vi "Unicode Tab Page Example.vi"() -> ()   [LabVIEW 2020]
doc: "This example demonstrates how to configure a new tab control to display unicode text."
uses:
  Unicode/Controls/String Encoding.ctl
  Types/UTF-8 String/UTF-8 String.lvclass/UTF-8 String.ctl
  Dialog & User Interface/Polymorphic VIs/Write Control Text/Write Tab Pages (UTF-8 String).vi
  Dialog & User Interface/Polymorphic VIs/Write Control Text/Write String Value (UTF-8 String).vi
  Unicode/Encode String.vi
  Dialog & User Interface/Polymorphic VIs/Write Control Text/Write Tab Pages (UTF-8 String).vi/5206cb6b-04fb-41f5-a37e-29c14f142303.vi
  Dialog & User Interface/Polymorphic VIs/Write Control Text/Write String Value (UTF-8 String).vi/5206cb6b-04fb-41f5-a37e-29c14f142303.vi
  Unicode/Detect String Encoding.vi
  Private/Conversion/Text to UTF-8.vi
  Private/Conversion/Polymorphic VIs/Text to UTF-8 (LabVIEW String).vi
  Private/Conversion/Encoded UTF-8 String to Encoded UTF-16LE String.vi
  Unicode/SubVIs/UTF-16 Byte Swap.vi
  Private/Conversion/UTF-8 to Text.vi
  Private/Conversion/Polymorphic VIs/UTF-8 to Text (LabVIEW String).vi
  Private/Conversion/Encoded UTF-16LE String to Encoded UTF-8 String.vi
  Unicode/Prepend BOM.vi
  Private/Conversion/Text as Encoded String.vi
  Private/Conversion/Polymorphic VIs/Text as Encoded String (UTF-8 String).vi
  Unicode/Strip BOM.vi
  Unicode/Detect String Encoding.vi/f4e2713d-ca87-487a-b901-d606fc3002c3.vi
  Unicode/SubVIs/Byte Order Marks.vi
  Unicode/Detect BOM.vi
  Types/UTF-8 String/Read Encoded UTF-8 String.vi
  Private/Library/gu_is_text_utf16.vi
  Private/Library/gu_is_text_utf8.vi
  Private/User Interface/Write String.vi
  Private/User Interface/Write Tab Control.vi
  Types/UTF-8 String/UTF-8 String.lvclass
  G-Unicode.lvlib
panel:
  in  "Tab Control":enum32{"Page 1", "Page 2", "Page 3", "Page 4"}(tab)
  out "Unicode String":string
  # "This example demonstrates how to configure a new tab control to display unicode text.\n\nWhen a tab control is first created the tab page text is not enabled for unicode display. To enable unicode display each page must first set the Independent Label property to TRUE. Once set, unicode text then needs to be copied over the text of every tab page. Once these steps have been carried out, the tab page text can then be programmatically written to using Write Control Text.vi and the desired unicode text.\n\nFollow the steps below to enable unicode text display for tab pages. Additional tab pages will also require running through these steps. Once unicode is enabled in each tab page, the VI can be saved and the unicode setting will persist.\n\n1. Run the VI. It will attempt to write unicode text to the tab pages, and at the same time will set the page's Independent Label property to TRUE. Note that the tab text will look wrong at this stage.\n2. Copy and paste the text from the Unicode String control to every tab page. This will enable unicode display.\n    - If this was done without having set Independent Label, LabVIEW might display a warning message (see below).\n3. Run the VI again. Now that unicode display is enabled on each tab page, unicode text can be programmatically written and displayed."
  # "Warning message displayed by LabVIEW when attempting to paste unicode text and Independent Label is FALSE."
  # "G"
  # "-Unicode"
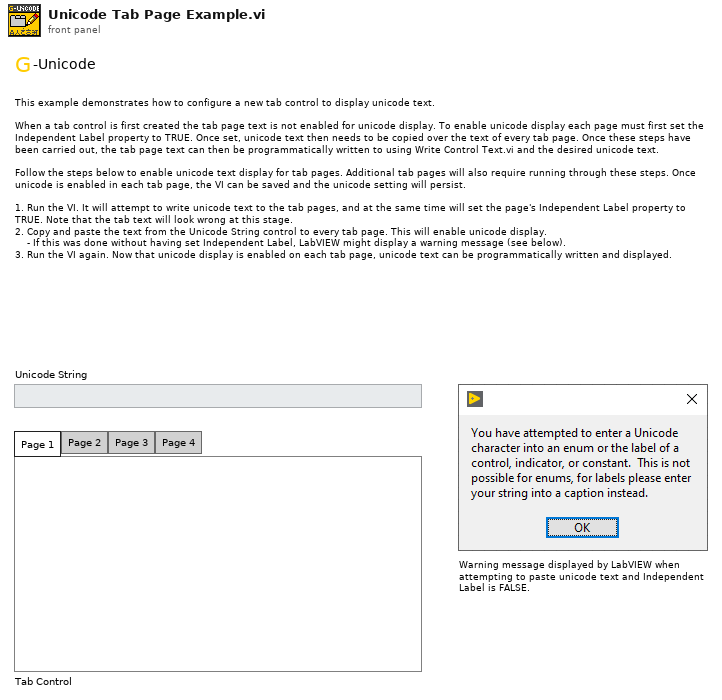
[diagram p1: front panel]
types:
  T1 = typedef "G-Unicode.lvlib/String Encoding.ctl" = enum16{"ANSI", "UTF-8", "UTF-16LE", "UTF-16BE", "Unknown"}
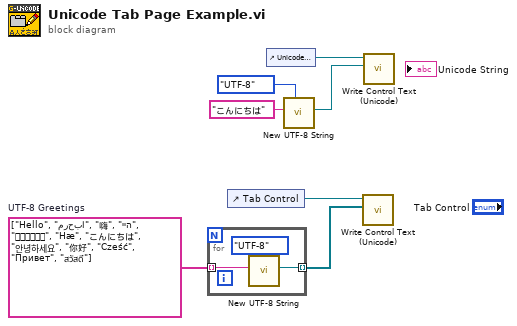
[diagram p0: block diagram]
diagram:
  w4 = string[] ["Hello", "مرحبا", "嗨", "היי", "नमस्ते", "Hæ", "こんにちは", "안녕하세요", "你好", "Cześć", "Привет", "สวัสดี"]  # UTF-8 Greetings
  n1 = for {
    tunnel: w4 -> [w10] mode=indexing
    tunnel: [w8] -> w3 mode=indexing
    n2 = call "New UTF-8 String.vi"("Input Encoding (ANSI)"=String_Encoding."UTF-8", "String"=w10) -> ("UTF-8 String"=w8:refnum<class "UTF-8 String.lvclass">)  [unwired: 8 in, 1 out]
  }
  n3 = control-ref of="Tab Control"() -> (w1:refnum<vi>)
  n4 = control-ref of="Unicode String"() -> (w2:refnum<vi>)
  n5 = call "New UTF-8 String.vi"("Input Encoding (ANSI)"=String_Encoding."UTF-8", "String"="こんにちは") -> ("UTF-8 String"=w7:refnum<class "UTF-8 String.lvclass">)  [unwired: 8 in, 1 out]
  n6 = call-poly "Write Control Text (Unicode).vi"("Value"=w3, "Control Ref"=w1) -> ()  [unwired: 9 in, 1 out]
  n7 = call-poly "Write Control Text (Unicode).vi"("Value"=w7, "Control Ref"=w2) -> ()  [unwired: 9 in, 1 out]
